vi "Scan for Tags.vi"(7 "Blacklist":string[](array[string]), 8 "error in (no error)":errorcluster, 11 "Variable Containers":refnum<k21>[](array[refnum])) -> (0 "error out":errorcluster, 1 "Top Level Folders Out":T1[](array[typedef]), 3 "Sync Tag Array":refnum<class "Synchronised Tag.lvclass">[](array[class]), 5 "Number of Tags":i32)   [LabVIEW 2016]
doc: "Scan the libraries for tags that can be loaded as synchronised tags and create the objects."
uses:
  Controls/Folders to Add.ctl
  Sync Tag Class/Synchronised Tag.lvclass
  Controls/Node Type.ctl
  <resource>/objmgr/ni.var.rc
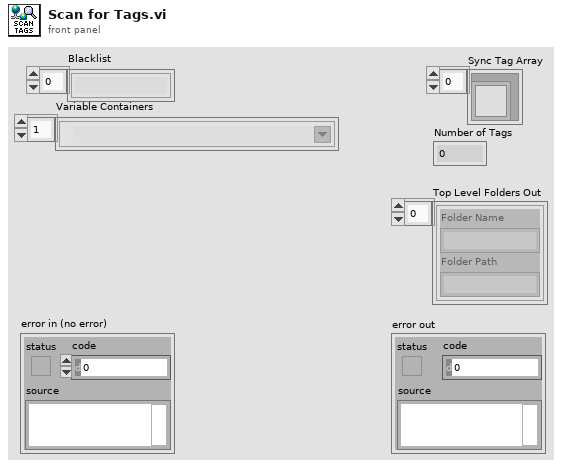
[diagram p1: front panel]
types:
  T1 = typedef "Folders to Add.ctl" = cluster{"Folder Name":string, "Folder Path":string}
  T2 = typedef "Node Type.ctl" = enum16{"Property", "Item", "Folder"}
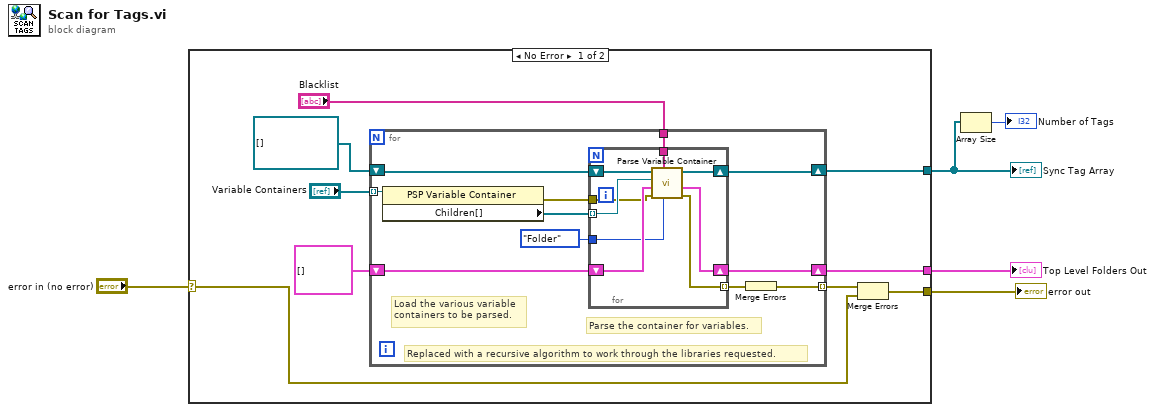
[diagram p0: block diagram]
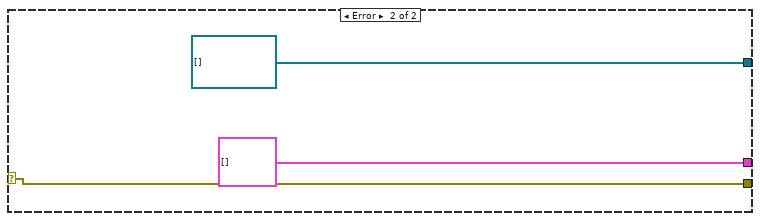
[diagram p2: hidden frame]
diagram:
  n1 = case shown="No Error" "error in (no error)" {
    selector: "error in (no error)" -> [w9 w37]
    tunnel: [w6 refnum<class "Synchronised Tag.lvclass">[] [] ("Tag Array In")] -> w2
    tunnel: [w12 T1[] [] ("Top Level Folders Out")] -> w3
    tunnel: [w10 w37] -> w5
    frame No Error {
      n2 = for {
        shift-right: [w25] -> w6
        shift-left: refnum<class "Synchronised Tag.lvclass">[] [] ("Tag Array In") -> [w24]
        tunnel: "Variable Containers" -> [w23] mode=indexing
        tunnel: "Blacklist" -> [w22]
        shift-right: [w20] -> w12
        shift-left: T1[] [] ("Top Level Folders Out") -> [w21]
        tunnel: [w19] -> w11 mode=indexing
        # "Parse the container for variables."
        # "Load the various variable\ncontainers to be parsed."
        # "Replaced with a recursive algorithm to work through the libraries requested."
        n3 = property class="PSP Variable Container"(reference=w23) -> (error out=w15:errorcluster, "Children[]"=w18:refnum<k21>[])  [unwired: 1 in, 1 out]
        n4 = for {
          shift-right: [w33] -> w25
          shift-left: w24 -> [w34]
          tunnel: Node_Type."Folder" ("Node Type") -> [w31]
          shift-right: [w30] -> w20
          shift-left: w21 -> [w32]
          tunnel: w18 -> [w29] mode=indexing
          tunnel: w22 -> [w28]
          tunnel: [w27] -> w16 mode=indexing
          tunnel: w15 -> [w26]
          n5 = call "Parse Variable Container.vi"("Parent Type"=w31, "Blacklist"=w28, "error in (no error)"=w26, "Top Level Folders in"=w32, "Variable Object"=w29, "Tag Array In"=w34) -> ("Error Out"=w27:errorcluster, "Top Level Folders Out"=w30:T1[], "Tag Array Out"=w33:refnum<class "Synchronised Tag.lvclass">[])  [unwired: 3 in]
        }
        n6 = Merge Errors(w16) -> (w19:errorcluster)
      }
      n7 = Merge Errors(w11, w9) -> (w10:errorcluster)
    }
    frame Error {
    }
  }
  "error out" <- w5
  "Top Level Folders Out" <- w3
  "Sync Tag Array" <- w2
  n8 = Array Size(array=w2) -> (size(s)=→"Number of Tags":i32)
